vi "SCD - Log Lyot Voltage Information.vi"(8 "error in (no error)":errorcluster, 10 "array":dbl[][](array[numeric]) format="%#.4g") -> (0 "error out":errorcluster)   [LabVIEW 2014]
doc: "Use this template to build a VI to use as a subVI."
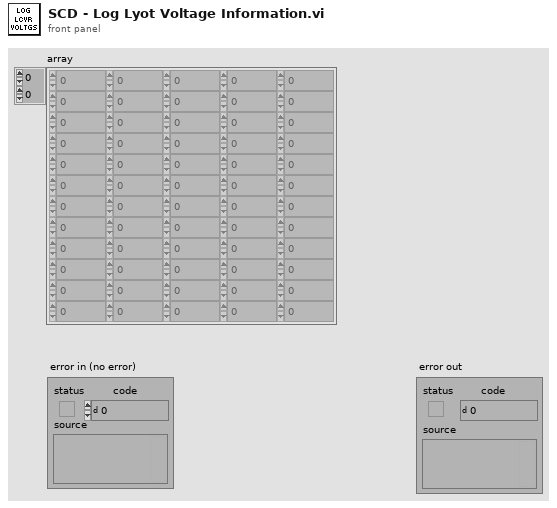
[diagram p1: front panel]
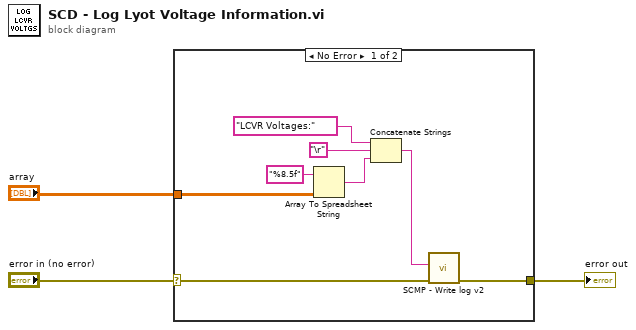
[diagram p0: block diagram]
diagram:
  n1 = case shown="No Error" "error in (no error)" {
    selector: "error in (no error)" -> [w6 w12]
    tunnel: [w5 w12] -> w2
    tunnel: "array" -> [w4 _]
    frame No Error {
      n2 = Array To Spreadsheet String(array=w4, 3:"%8.5f" ("format string")) -> (spreadsheet string=w8:string)  [unwired: 1 in]
      n3 = Concatenate Strings("LCVR Voltages:" ("string"), "\r", w8) -> (w7:string)
      n4 = call "SCMP - Write log v2.vi"("Error to log"=w6, "data"=w7) -> ("error out"=w5:errorcluster)  [unwired: 7 in, 2 out]
    }
    frame Error {
    }
  }
  "error out" <- w2
